vi "Ex. 2 Block diagram functions.vi"() -> ()   [LabVIEW 2024]
panel:
  out "a-b":dbl
  in  "b":dbl=7.0
  out "a+b":dbl
  in  "a":dbl=12.0
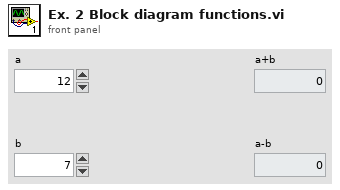
[diagram p1: front panel]
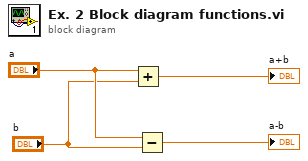
[diagram p0: block diagram]
diagram:
  n1 = Add(x="a", y="b") -> (x+y=→"a+b":dbl)
  n2 = Subtract(x="a", y="b") -> (x-y=→"a-b":dbl)
